vi "PythonNode_ConcatenateTwoStrings.vi"() -> ()   [LabVIEW 2019]
doc: "This example demonstrates how to call a Python function and pass strings as arguments. It uses a python function to concatenate two strings."
uses:
  support/PythonVersionsEnum.ctl
panel:
  out "concatenated string":string
  in  "str2":string="World"
  in  "str1":string="Hello "
  out "error out":errorcluster
  in  "error in (no error)":errorcluster
  in  "python version":T1
  # "Overview: Demonstrates how to call a Python function and pass strings as arguments.\nRequirements: Python 2.7 or 3.6 with the same bitness as LabVIEW.\nInstructions:\n1. Set the Python version to the version of Python you want to execute code in.\n2. Run the VI. You should see the result of concatenating \"str1\" and \"str2\" in the indicator \"concatenated string\".\n3. See comments on the block diagram of this VI and in \"ExamplePythonModule.py\" for more information about how the call python node passes arguments and handles return values."
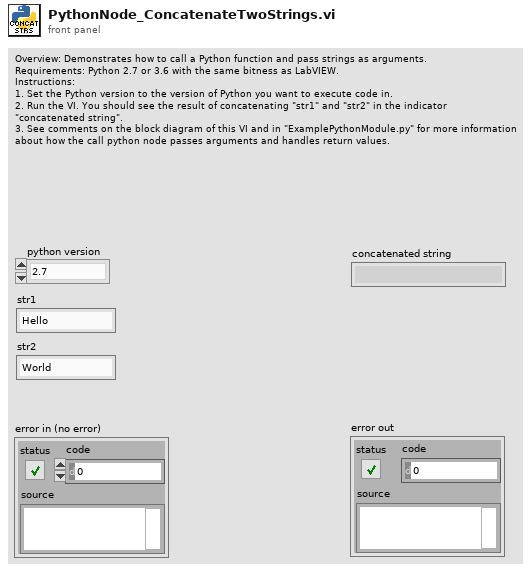
[diagram p1: front panel]
types:
  T1 = typedef "PythonVersionsEnum.ctl" = enum16{"2.7", "3.6"}
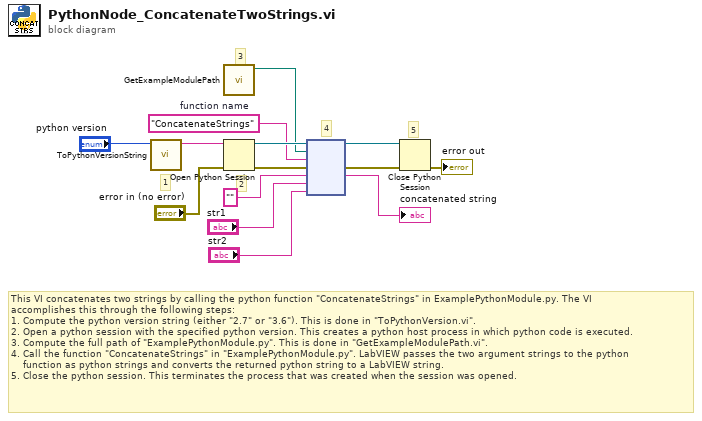
[diagram p0: block diagram]
diagram:
  w8 = "ConcatenateStrings"  # function name
  # "5"
  # "4"
  # "2"
  # "3"
  # "1"
  # "This VI concatenates two strings by calling the python function \"ConcatenateStrings\" in ExamplePythonModule.py. The VI\naccomplishes this through the following steps:\n1. Compute the python version string (either \"2.7\" or \"3.6\"). This is done in \"ToPythonVersion.vi\". \n2. Open a python session with the specified python version. This creates a python host process in which python code is executed.\n3. Compute the full path of \"ExamplePythonModule.py\". This is done in \"GetExampleModulePath.vi\".\n4. Call the function \"ConcatenateStrings\" in \"ExamplePythonModule.py\". LabVIEW passes the two argument strings to the python\n    function as python strings and converts the returned python string to a LabVIEW string.\n5. Close the python session. This terminates the process that was created when the session was opened."
  n1 = call "ToPythonVersionString.vi"("python version"="python version") -> ("python version string"=w14:string)  [unwired: 10 in]
  n2 = call "GetExampleModulePath.vi"() -> ("module path"=w9:path)  [unwired: 11 in]
  n3 = Open Python Session(python version=w14, 3:"error in (no error)") -> (session out=w11:refnum<k35>, error out=w10:errorcluster)  [unwired: 1 in]
  n4 = node(w11, w9, w8, w10, "" ("str1"), "str1", "str2") -> (w7:refnum<k35>, w6:errorcluster, →"concatenated string":string)  [unwired: 2 in, 2 out]
  n5 = Close Python Session(session in=w7, error in=w6) -> (11:→"error out":errorcluster)
